vi "CRYUnflatten Signal Generator.vi"(11 "Flat Signal Gen'r settings":string="%#_6p") -> (0 "Error?":bool=TRUE, 2 "Signal Gen'r settings":T1={"gen'r mode"=0, "frequency"=0, "output level"=0.0, "wave path"="", "wav play mode"=0, "duration"=0.0, "n times"=0, "channel"=0, "wav level"=0.0, "EQ"=FALSE, "f knob log"=FALSE, "f knob low"=0.0, "f knob high"=0.0, "ol knob log"=FALSE, "ol knob low"=0.0, "ol knob high"=0.0, "Lin Display Prefs"="%#_6p", "dB Display Prefs"="%.1f", "Duration noise"=20.0, "Min freq noise"=20.0, "Max freq noise"=20000.0, "Channel String"="", "Play Sine Wave"=0} {"Duration noise" format="%.2f"; "Max freq noise" format="%.2f"; "Min freq noise" format="%.2f"; "ol knob high" format="%.2f"; "ol knob low" format="%.2f"; "f knob high" format="%.2f"; "f knob low" format="%.2f"; "wav level" format="%.2f"; "duration" format="%.2f"; "output level" format="%.2f"}, 3 "Header info":T2={"Data type"="Data            ", "Version"=1, "Dimensions"=0})   [LabVIEW 2013]
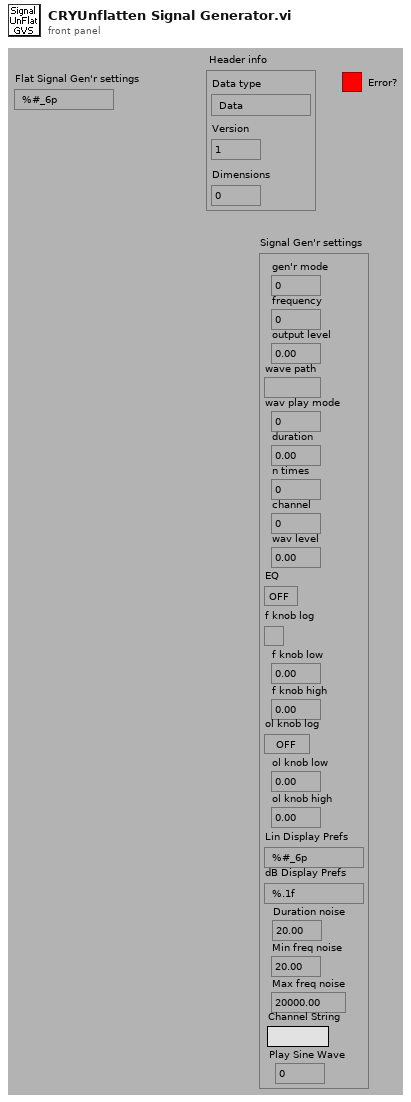
[diagram p1: front panel]
types:
  T1 = cluster{"gen'r mode":i32, "frequency":u32, "output level":dbl, "wave path":string, "wav play mode":i32, "duration":dbl, "n times":i32, "channel":i32, "wav level":dbl, "EQ":bool, "f knob log":bool, "f knob low":dbl, "f knob high":dbl, "ol knob log":bool, "ol knob low":dbl, "ol knob high":dbl, "Lin Display Prefs":string, "dB Display Prefs":string, "Duration noise":dbl, "Min freq noise":dbl, "Max freq noise":dbl, "Channel String":string, "Play Sine Wave":i32}
  T2 = cluster{"Data type":string, "Version":u16, "Dimensions":u8}
  T3 = cluster{"unsigned byte array[0]":u8, "unsigned byte array[1]":u8, "unsigned byte array[2]":u8}
  T4 = cluster{"substring":string, u16, "unsigned byte array[2]":u8}
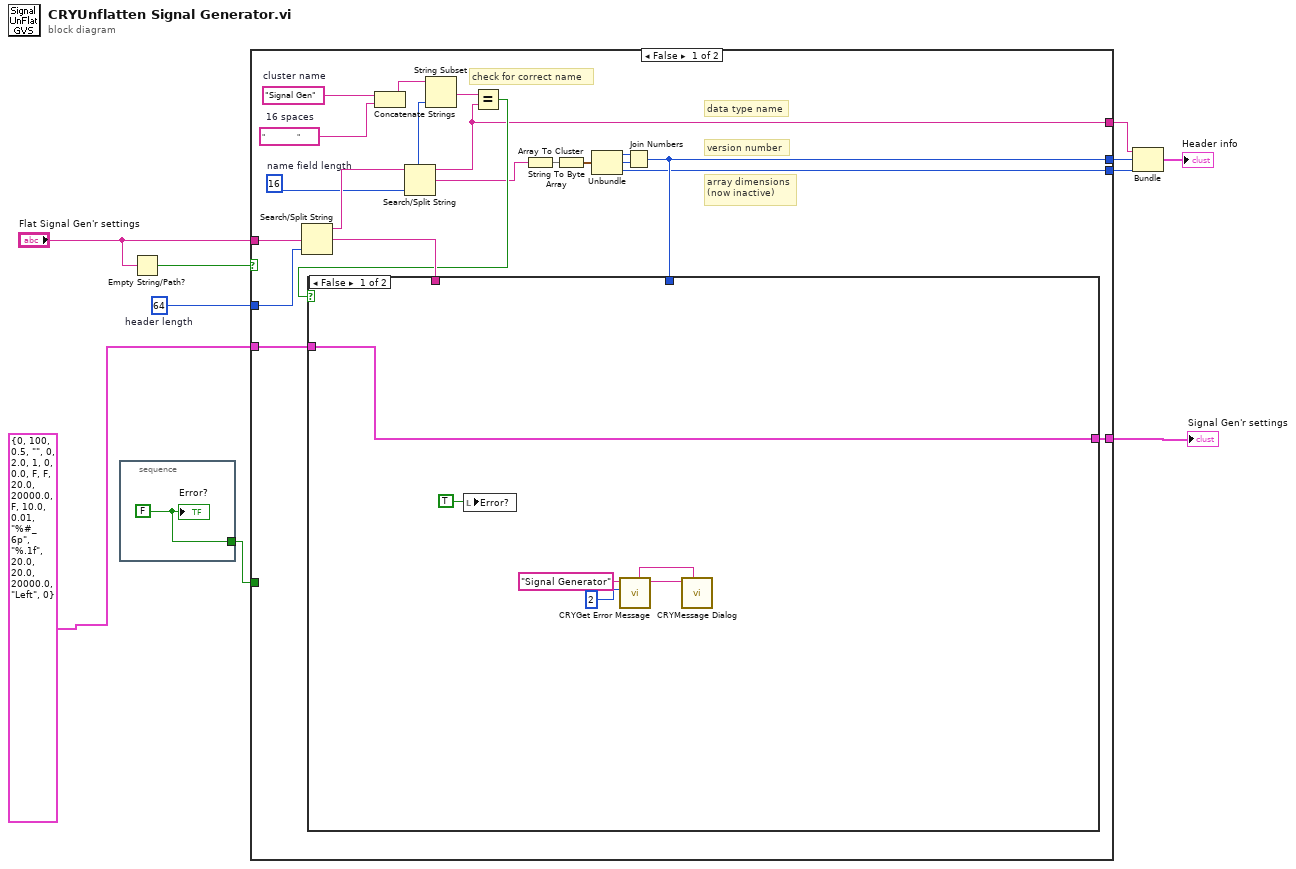
[diagram p0: block diagram]
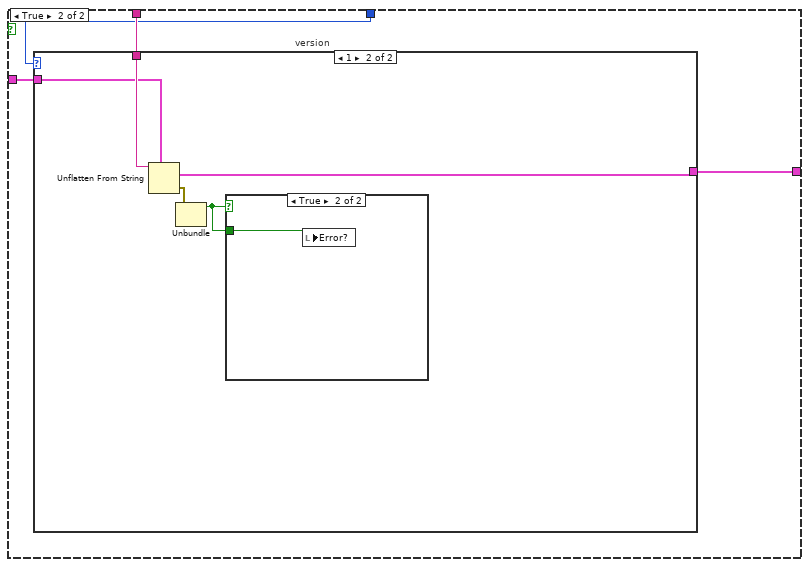
[diagram p2: hidden frame]
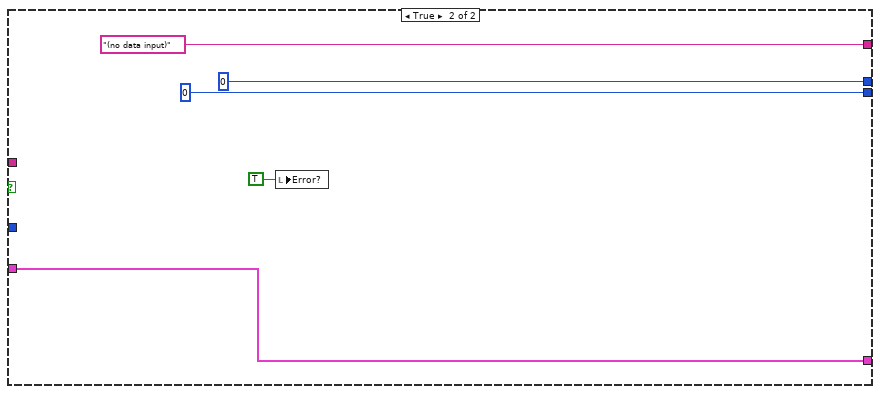
[diagram p5: hidden frame]
diagram:
  w9 = 64  # header length
  n1 = stacked-sequence {
    tunnel: [w11] -> w5
    frame #0 {
      w11 = FALSE
      "Error?" <- w11
    }
  }
  n2 = Empty String/Path?(string/path="Flat Signal Gen'r settings") -> (empty?=w10:bool)
  n3 = case shown="False" w10 {
    tunnel: "Flat Signal Gen'r settings" -> [w31 _]
    tunnel: w9 -> [w25 _]
    tunnel: [w22 u16 0] -> w7
    tunnel: [w15 u8 0] -> w8
    tunnel: [w16 "(no data input)" ("substring")] -> w6
    tunnel: w5 -> [_ _]
    tunnel: [w14 w49] -> w2
    tunnel: T1 {"gen'r mode"=0, "frequency"=100, "output level"=0.5, "wave path"="", "wav play mode"=0, "duration"=2.0, "n times"=1, "channel"=0, "wav level"=0.0, "EQ"=FALSE, "f knob log"=FALSE, "f knob low"=20.0, "f knob high"=20000.0, "ol knob log"=FALSE, "ol knob low"=10.0, "ol knob high"=0.01, "Lin Display Prefs"="%#_6p", "dB Display Prefs"="%.1f", "Duration noise"=20.0, "Min freq noise"=20.0, "Max freq noise"=20000.0, "Channel String"="Left", "Play Sine Wave"=0} ("Signal Gen'r settings") -> [w13 w49]
    frame False {
      w12 = "Signal Gen"  # cluster name
      w20 = "                "  # 16 spaces
      w18 = 16  # name field length
      # "check for correct name"
      # "array dimensions\n(now inactive)"
      # "version number"
      # "data type name"
      n4 = Search/Split String(string=w31, offset (0)=w25) -> (substring before match=w24:string, match + rest of string=w26:string)  [unwired: 2 out]
      n5 = Concatenate Strings(w12, w20) -> (w19:string)
      n6 = Search/Split String(string=w24, offset (0)=w18) -> (substring before match=w16:string, match + rest of string=w21:string)  [unwired: 2 out]
      n7 = String Subset(string=w19, length (rest)=w18) -> (substring=w17:string)  [unwired: 1 out]
      n8 = Equal?(x=w17, y=w16) -> (x = y?=w23:bool)
      n9 = String To Byte Array(string=w21) -> (unsigned byte array=w30:u8[])
      n10 = Array To Cluster(array=w30) -> (cluster=w29:T3)
      n11 = Unbundle(w29) -> ("unsigned byte array[0]"=w28:u8, "unsigned byte array[1]"=w27:u8, "unsigned byte array[2]"=w15:u8)
      n12 = Join Numbers(hi=w28, lo=w27) -> ((hi.lo)=w22:u16)
      n13 = case shown="False" w23 {
        tunnel: w26 -> [_ w41]
        tunnel: w22 -> [_ w40]
        tunnel: [w36 w39] -> w14
        tunnel: w13 -> [w36 w38]
        frame False {
          n14 = local write "Error?"(TRUE) -> ()
          n15 = call "CRYGet Error Message.vi"("Error No"=2, "Kind"="Signal Generator") -> ("Message"=w33:string, "Window Title"=w32:string)  [unwired: 4 in, 4 out]
          n16 = call "CRYMessage Dialog.vi"("Window Title"=w32, "Message Content"=w33) -> ()  [unwired: 8 in, 2 out]
        }
        frame True {
          n17 = case "version" shown="1" w40 {
            tunnel: w41 -> [_ w47]
            tunnel: [w42 w43] -> w39
            tunnel: w38 -> [w42 w44]
            frame Default {
            }
            frame 1 {
              n18 = Unflatten From String(type=w44, binary string=w47) -> (value=w43:T1, error out=w45:errorcluster)  [unwired: 1 in, 3 out]
              n19 = Unbundle(w45) -> ("status"=w46:bool)  [unwired: 2 out]
              n20 = case shown="True" w46 {
                tunnel: w46 -> [_ w48]
                frame False {
                }
                frame True {
                  n21 = local write "Error?"(w48) -> ()
                }
              }
            }
          }
        }
      }
    }
    frame True {
      n22 = local write "Error?"(TRUE ("Error?")) -> ()
    }
  }
  "Signal Gen'r settings" <- w2
  n23 = Bundle("substring"=w6, w7, "unsigned byte array[2]"=w8) -> (→"Header info":T4)  [unwired: 1 out]
